vi "DutyM1.vi"(7 "Duty":i16 max=127 step=1, 8 "error in (no error)":errorcluster, 10 "Address":u8, 11 "VISA Refnum in":refnum<visa-resource-name>) -> (0 "error out":errorcluster, 2 "Valid":bool, 3 "VISA Refnum out":refnum<visa-resource-name>)   [LabVIEW 2015, in "Ion Motion Roboclaw.lvlib"]
uses:
  <instrlib>/Ion Motion Roboclaw/Ion Motion Roboclaw.lvlib
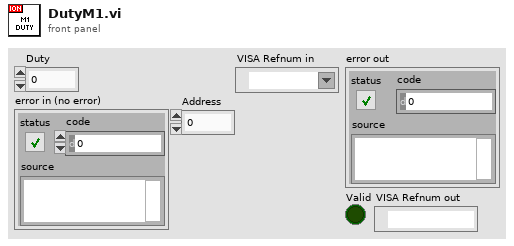
[diagram p1: front panel]
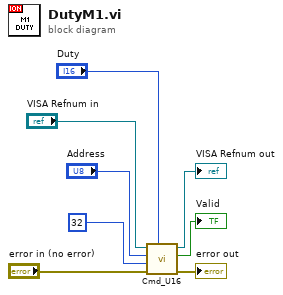
[diagram p0: block diagram]
diagram:
  n1 = call <instrlib>:"Cmd_U16.vi"("Argument"="Duty", "error in (no error)"="error in (no error)", "Cmd"=u8 32, "Address"="Address", "VISA Refnum in"="VISA Refnum in") -> ("error out"=→"error out":errorcluster, "Valid"=→"Valid":bool, "VISA Refnum out"=→"VISA Refnum out":refnum<visa-resource-name>)  [unwired: 4 in]
